vi "Action on Compile.vi"(8 "error in (no error)":errorcluster, 11 "Device Ref in":T1=18446744073709551615 format="%.0x") -> (0 "error out":errorcluster)   [LabVIEW 2013, in "Modbus System Explorer.lvlib"]
uses:
  Modbus System Explorer.lvlib
  <vilib>/NI Veristand/Custom Device API/Custom Device Item Ref.ctl
  Shared/Channels Ref.ctl
  Shared/FIFO Indexes.ctl
  <vilib>/NI Veristand/Custom Device API/Custom Device Channel Type.ctl
  Glyphs/Modbus Property Names.vi
  <vilib>/NI Veristand/Custom Device API/Get Item Property (Variant).vi
  <vilib>/NI Veristand/Custom Device API/Set Item Property (Variant).vi
  Shared/Modbus Shared.lvlib
  <vilib>/NI Veristand/Custom Device API/Custom Device API.lvlib
  <vilib>/NI Veristand/Custom Device Tools/Custom Device Utility Library/Custom Device Utility Library.lvlib
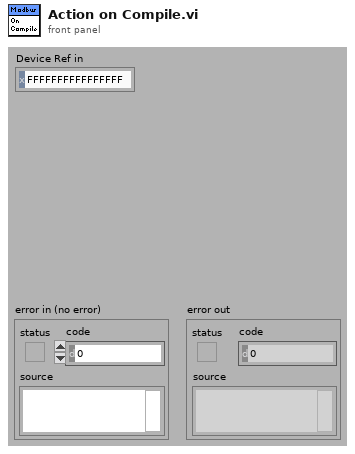
[diagram p1: front panel]
types:
  T1 = typedef "Custom Device API.lvlib/Custom Device Item Ref.ctl" = u64
  T2 = typedef "Modbus Shared.lvlib/Channels Ref.ctl" = cluster{"Array of Refs":T1[]}
  T3 = cluster{"status":bool, "code":i32, "source 2":string}
  T4 = typedef "Modbus Shared.lvlib/FIFO Indexes.ctl" = cluster{"FIFO Indexes":i32[], "FIFO Buffer":T5}
  T5 = typedef "Custom Device API.lvlib/Custom Device Channel Type.ctl" = enum16{"Input", "Output"}
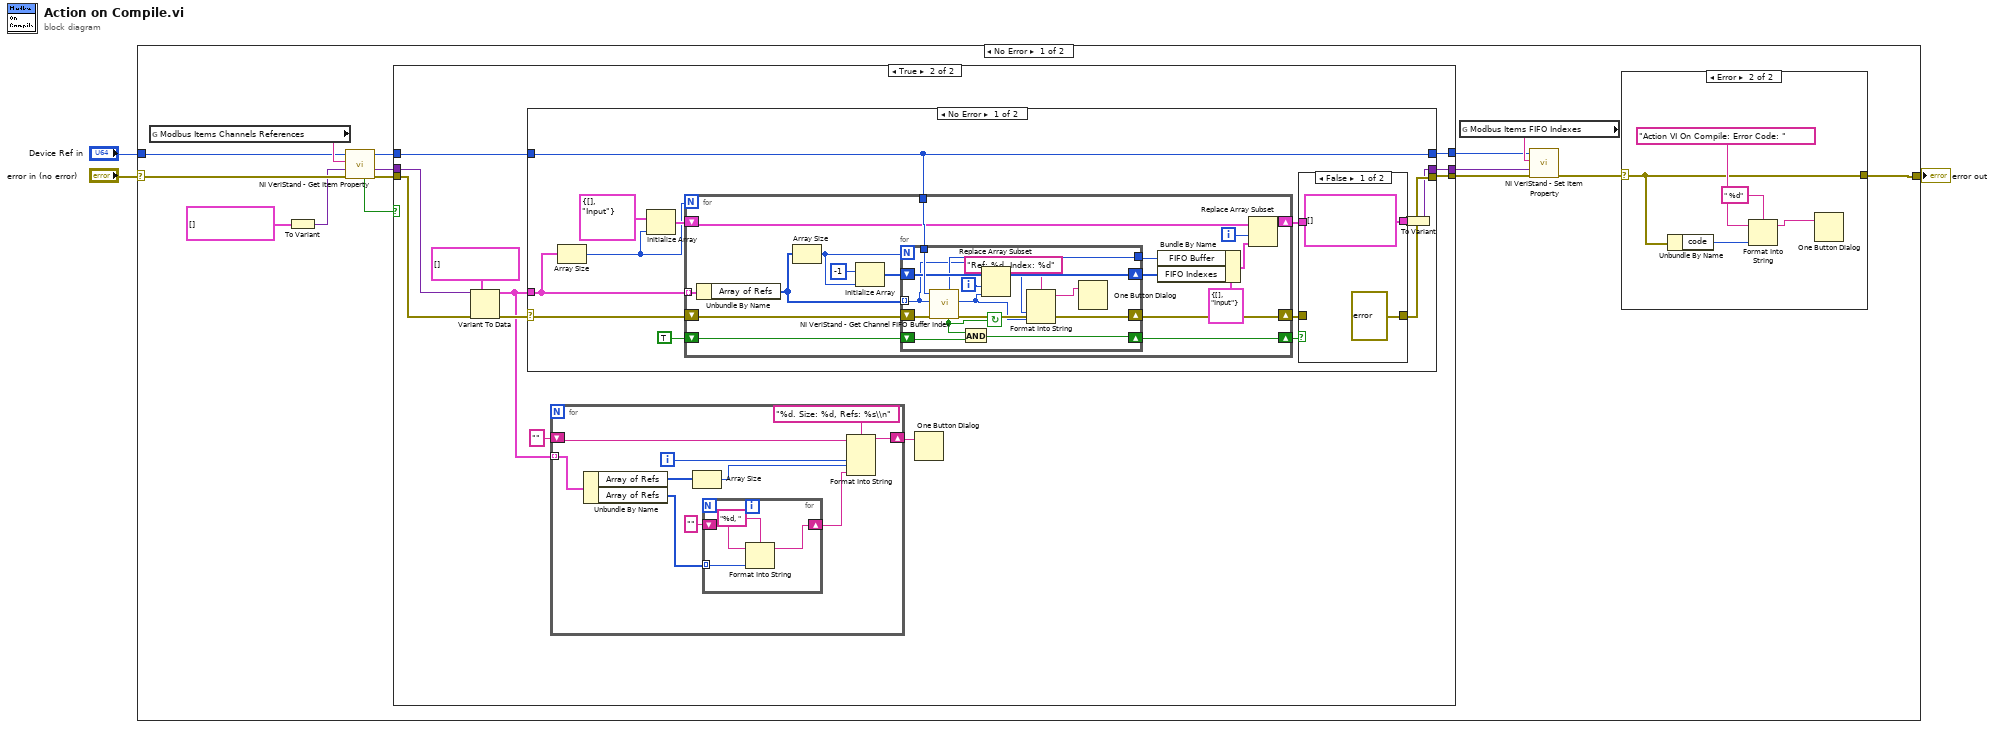
[diagram p0: block diagram]
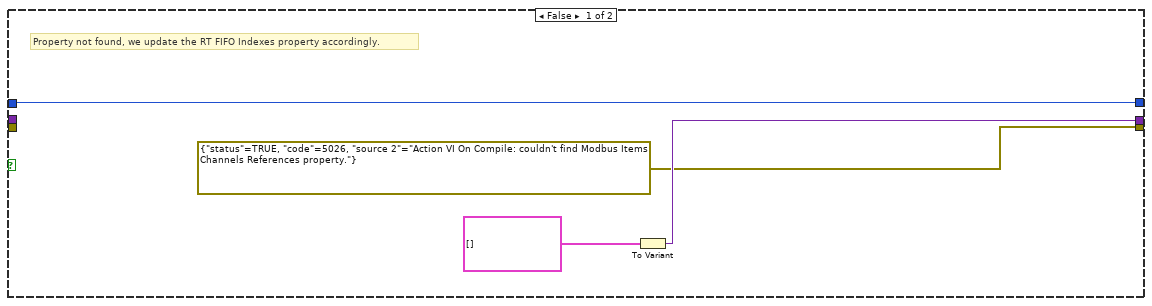
[diagram p3: hidden frame]
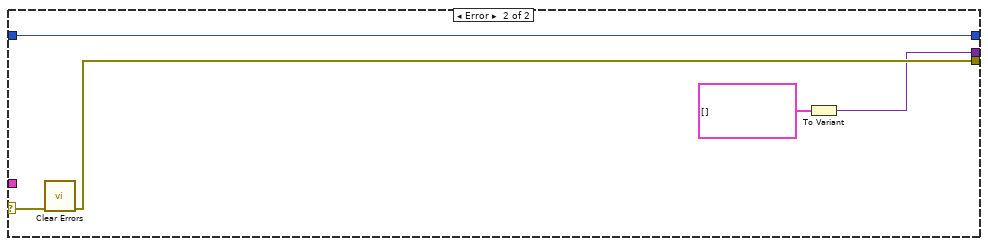
[diagram p5: hidden frame]
diagram:
  n1 = case shown="No Error" "error in (no error)" {
    selector: "error in (no error)" -> [w16 w107]
    tunnel: [w4 w107] -> w3
    tunnel: "Device Ref in" -> [w17 _]
    frame No Error {
      n2 = global read "Modbus Property Names.vi" "Modbus Items Channels References"() -> (w18:string)
      n3 = To Variant(anything=T2[] []) -> (Variant=w14:variant)
      n4 = call-poly <vilib>:"NI VeriStand - Get Item Property.vi"("error in (no error)"=w16, "Default Value"=w14, "Property Name"=w18, "Item Ref in"=w17) -> ("error out"=w11:errorcluster, "Value"=w13:variant, "Item Ref out"=w10:T1, "Found?"=w12:bool)  [unwired: 4 in]
      n5 = case shown="True" w12 {
        tunnel: w13 -> [_ w39]
        tunnel: w11 -> [_ w38]
        tunnel: w10 -> [w26 w35]
        tunnel: [T3 {"status"=TRUE, "code"=5026, "source 2"="Action VI On Compile: couldn't find Modbus Items Channels References property."} ("error IO") w34] -> w8
        tunnel: [w26 w33] -> w7
        tunnel: [w27 w32] -> w6
        frame False {
          # "Property not found, we update the RT FIFO Indexes property accordingly."
          n6 = To Variant(anything=T4[] []) -> (Variant=w27:variant)
        }
        frame True {
          n7 = Variant To Data(error in=w38, type=T2[] [], Variant=w39) -> (data=w30:T2[], error out=w36:errorcluster)
          n8 = case shown="No Error" w36 {
            selector: w36 -> [w61 w106]
            tunnel: w30 -> [w64 _]
            tunnel: w35 -> [w62 w105]
            tunnel: [w62 w105] -> w33
            tunnel: [w57 w104] -> w34
            tunnel: [w54 w102] -> w32
            frame No Error {
              n9 = Array Size(array=w64) -> (size(s)=w63:i32)
              n10 = Initialize Array(T4 {"FIFO Indexes"=[], "FIFO Buffer"=enum."Input"} ("Cluster"), w63) -> (w65:T4[])
              n11 = for {
                N: w63 -> [_]
                tunnel: w62 -> [w87]
                shift-right: [w85] -> w56
                shift-left: w65 -> [w86]
                tunnel: w64 -> [w81] mode=indexing
                shift-right: [w74] -> w58
                shift-left: w61 -> [w79]
                shift-right: [w71] -> w59
                shift-left: TRUE -> [w72]
                i -> [w84]
                n12 = Unbundle By Name(w81) -> ("Array of Refs"=w80:T1[])
                n13 = Array Size(array=w80) -> (size(s)=w77:i32)
                n14 = Initialize Array(-1, w77) -> (w76:i32[])
                n15 = for {
                  N: w77 -> [_]
                  tunnel: w87 -> [w101]
                  tunnel: w80 -> [w91] mode=indexing
                  shift-right: [w98] -> w75
                  shift-left: w76 -> [w99]
                  shift-right: [w96] -> w74
                  shift-left: w79 -> [w100]
                  tunnel: [w95] -> w73
                  shift-right: [w92] -> w71
                  shift-left: w72 -> [w93]
                  i -> [w97]
                  stop <- w94 continue-if-true
                  n16 = call <vilib>:"NI VeriStand - Get Channel FIFO Buffer Index.vi"("error in"=w100, "Channel Ref"=w91, "Device Ref in"=w101) -> ("error out"=w96:errorcluster, "Channel FIFO Buffer Index"=w90:i32, "Found"=w94:bool, "FIFO Buffer"=w95:T5)  [unwired: 4 in, 1 out]
                  n17 = And(x=w94, y=w93) -> (x .and. y?=w92:bool)
                  n18 = Replace Array Subset(array=w99, new element=w90, index=w97) -> (w98:i32[])
                  n19 = Format Into String(format string="Ref: %d  Index: %d", w91, w90) -> (resulting string=w89:string)  [unwired: 2 in, 1 out]
                  n20 = One Button Dialog(message=w89) -> ()  [unwired: 1 in, 1 out]
                }
                n21 = Bundle By Name(cluster=T4 {"FIFO Indexes"=[], "FIFO Buffer"=enum."Input"} ("Cluster"), "FIFO Buffer"=w73, "FIFO Indexes"=w75) -> (w83:T4)
                n22 = Replace Array Subset(array=w86, new element=w83, index=w84) -> (w85:T4[])
              }
              n23 = case shown="False" w59 {
                tunnel: w58 -> [_ w70]
                tunnel: [T3 {"status"=TRUE, "code"=5025, "source 2"="Action VI On Compile: couldn't find all FIFO Indexes."} ("error IO") w70] -> w57
                tunnel: w56 -> [_ w69]
                tunnel: [T4[] [] w69] -> w55
                frame False {
                }
                frame True {
                }
              }
              n24 = To Variant(anything=w55) -> (Variant=w54:variant)
            }
            frame Error {
              n25 = call <vilib>:"Clear Errors.vi"("error in (no error)"=w106) -> ("error out"=w104:errorcluster)  [unwired: 6 in]
              n26 = To Variant(anything=T4[] []) -> (Variant=w102:variant)
            }
          }
          n27 = for {
            tunnel: w30 -> [w47] mode=indexing
            shift-right: [w49] -> w29
            shift-left: "" -> [w48]
            i -> [w45]
            n28 = Unbundle By Name(w47) -> ("Array of Refs"=w44:T1[], "Array of Refs"=w41:T1[])
            n29 = Array Size(array=w44) -> (size(s)=w43:i32)
            n30 = for {
              shift-right: [w51] -> w40
              shift-left: "" -> [w52]
              tunnel: w41 -> [w53] mode=indexing
              n31 = Format Into String(format string="%d, ", initial string=w52, w53) -> (resulting string=w51:string)  [unwired: 1 in, 1 out]
            }
            n32 = Format Into String(format string="%d. Size: %d, Refs: %s\\n", initial string=w48, w45, w43, w40) -> (resulting string=w49:string)  [unwired: 1 in, 1 out]
          }
          n33 = One Button Dialog(message=w29) -> ()  [unwired: 1 in, 1 out]
        }
      }
      n34 = global read "Modbus Property Names.vi" "Modbus Items FIFO Indexes"() -> (w9:string)
      n35 = call-poly <vilib>:"NI VeriStand - Set Item Property.vi"("error in (no error)"=w8, "Value"=w6, "Property Name"=w9, "Item Ref in"=w7) -> ("error out"=w5:errorcluster)  [unwired: 5 in, 2 out]
      n36 = case shown="Error" w5 {
        selector: w5 -> [w19 w20]
        tunnel: [w19 w20] -> w4
        frame No Error {
        }
        frame Error {
          n37 = Unbundle By Name(w20) -> ("code"=w24:i32)
          n38 = Format Into String(format string=" %d", initial string="Action VI On Compile: Error Code: " ("message"), w24) -> (resulting string=w22:string)  [unwired: 1 in, 1 out]
          n39 = One Button Dialog(message=w22) -> ()  [unwired: 1 in, 1 out]
        }
      }
    }
    frame Error {
    }
  }
  "error out" <- w3
